vi "dfd_Reorganize Coef.vi"(9 "#phase in":i32, 11 "org coef":i32[](array[numeric])) -> (1 "#phase":i32, 2 "#taps per phase":i32, 3 "coef out":i32[](array[numeric]))   [LabVIEW 2017, in "NI_DigFilter_FXP.lvlib"]
uses:
  <vilib>/addons/Digital Filter Design/NI_DigFilter_FXP.lvlib
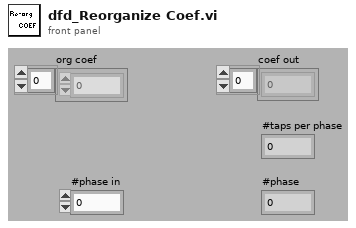
[diagram p1: front panel]
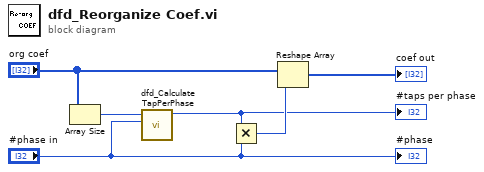
[diagram p0: block diagram]
diagram:
  n1 = Array Size(array="org coef") -> (size(s)=w3:i32)
  n2 = call <vilib>:"dfd_Calculate TapPerPhase.vi"("factor"="#phase in", "#taps"=w3) -> ("tapPerPhase"=w1:i32)  [unwired: 9 out]
  "#taps per phase" <- w1
  n3 = Multiply(x=w1, y="#phase in") -> (x*y=w5:i32)
  n4 = Reshape Array("org coef", w5) -> (→"coef out":i32[])
  "#phase" <- "#phase in"
